vi "CREATE ARCHIVE USER SQL QUERY.vi"(0 "What to Search":string, 5 "Search Column Name":string, 7 "Sorting Column Name":string, 9 "Column to Search In":u16, 12 "Date Range":u16(ring) items=["Greater Than", "Less Than", "Between"], 13 "Dates Less Than":string="8/1/2023", 14 "Dates Greater Than":string="8/1/2023") -> (4 "SQL QUERY":string)   [LabVIEW 2019]
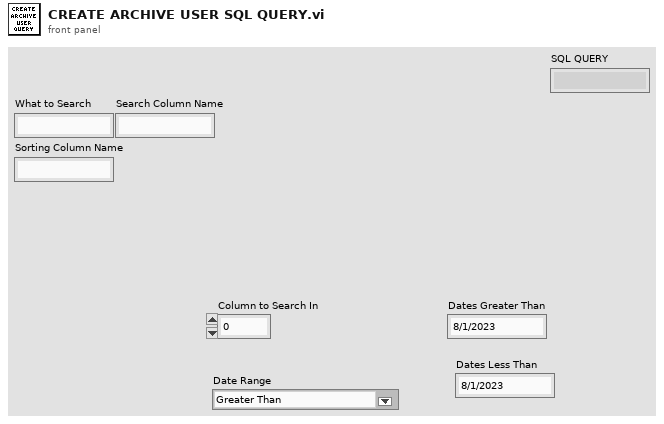
[diagram p1: front panel]
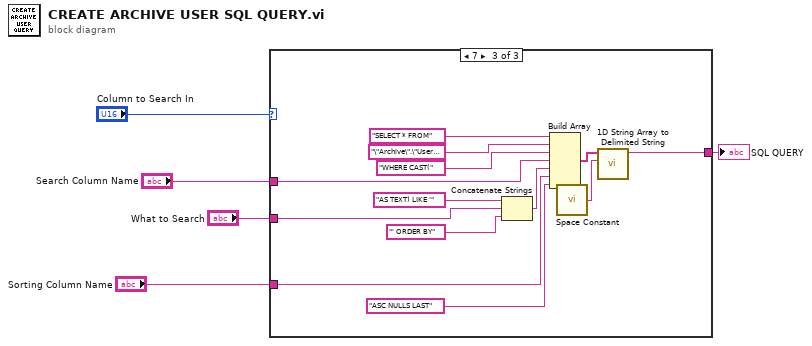
[diagram p0: block diagram]
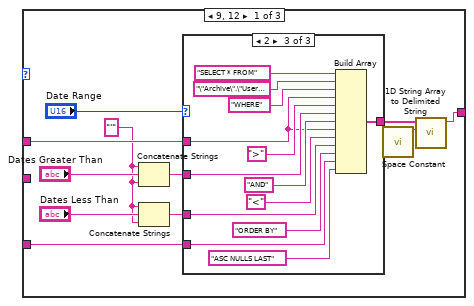
[diagram p2: hidden frame]
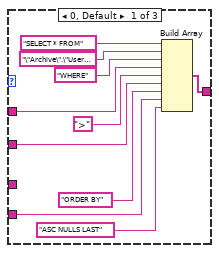
[diagram p3: hidden frame]
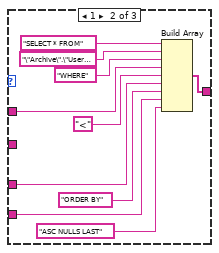
[diagram p4: hidden frame]
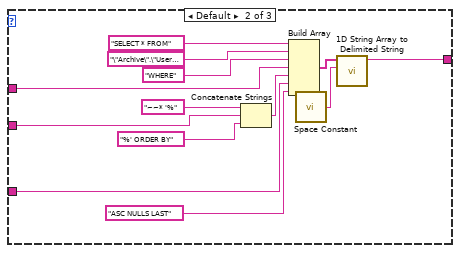
[diagram p5: hidden frame]
diagram:
  n1 = case shown="7" "Column to Search In" {
    tunnel: [w14 w56 w69] -> w5
    tunnel: "Sorting Column Name" -> [w11 w52 w65]
    tunnel: "Search Column Name" -> [w12 w51 w64]
    tunnel: "What to Search" -> [_ w50 w63]
    frame 9, 12 {
      w6 = "'"
      n2 = Concatenate Strings(w6, "Dates Greater Than", w6) -> (w10:string)
      n3 = Concatenate Strings(w6, "Dates Less Than", w6) -> (w9:string)
      n4 = case shown="2" "Date Range" {
        tunnel: [w23 w33 w46] -> w13
        tunnel: w12 -> [w22 w32 w42]
        tunnel: w10 -> [w20 _ w44]
        tunnel: w11 -> [w18 w29 w38]
        tunnel: w9 -> [_ w27 w40]
        frame 0, Default {
          n5 = Build Array("SELECT * FROM", "\"Archive\".\"Users\"" ("string"), "WHERE" ("string"), w22, ">" ("string"), w20, "ORDER BY" ("string"), w18, "ASC NULLS LAST" ("string")) -> (w23:string[])
        }
        frame 1 {
          n6 = Build Array("SELECT * FROM", "\"Archive\".\"Users\"" ("string"), "WHERE" ("string"), w32, "<" ("string"), w27, "ORDER BY" ("string"), w29, "ASC NULLS LAST" ("string")) -> (w33:string[])
        }
        frame 2 {
          n7 = Build Array("SELECT * FROM", "\"Archive\".\"Users\"" ("string"), "WHERE" ("string"), w42, ">" ("string"), w44, "AND" ("string"), w42, "<" ("string"), w40, "ORDER BY" ("string"), w38, "ASC NULLS LAST" ("string")) -> (w46:string[])
        }
      }
      n8 = call <vilib>:"Space Constant.vi"() -> ("String"=w15:string)
      n9 = call <vilib>:"1D String Array to Delimited String.vi"("delimiter"=w15, "string array"=w13) -> ("delimited string"=w14:string)  [unwired: 9 in]
    }
    frame Default {
      n10 = Concatenate Strings("~~* '%" ("string"), w50, "%' ORDER BY" ("string")) -> (w53:string)
      n11 = Build Array("SELECT * FROM", "\"Archive\".\"Users\"" ("string"), "WHERE" ("string"), w51, w53, w52, "ASC NULLS LAST" ("string")) -> (w58:string[])
      n12 = call <vilib>:"Space Constant.vi"() -> ("String"=w57:string)
      n13 = call <vilib>:"1D String Array to Delimited String.vi"("delimiter"=w57, "string array"=w58) -> ("delimited string"=w56:string)  [unwired: 9 in]
    }
    frame 7 {
      n14 = Concatenate Strings("AS TEXT) LIKE '" ("string"), w63, "' ORDER BY" ("string")) -> (w66:string)
      n15 = Build Array("SELECT * FROM", "\"Archive\".\"Users\"" ("string"), "WHERE CAST(" ("string"), w64, w66, w65, "ASC NULLS LAST" ("string")) -> (w71:string[])
      n16 = call <vilib>:"Space Constant.vi"() -> ("String"=w70:string)
      n17 = call <vilib>:"1D String Array to Delimited String.vi"("delimiter"=w70, "string array"=w71) -> ("delimited string"=w69:string)  [unwired: 9 in]
    }
  }
  "SQL QUERY" <- w5
